vi "AF_Configuration.vi"(1 "ClassRef/ClassPath(If empty Configuration default will be modified)":variant, 5 "Error In":errorcluster) -> (19 "Error Out":errorcluster)   [LabVIEW 2020]
uses:
  LvIcon_class/GDSLvIcon_ColorControl.ctl
  SubVIs/GOOP_WirePattern.ctl
  SubVIs/GOOP_HelpButton.ctl
  SubVIs/GOOP_WireConfigurationType.ctl
  AF_SettingsType.ctl
panel:
  in  "_MessageFolderName":string caption="Virtual message folder name to use"
  in  "_HelpDefaultConfiguration":T1
  in  "_Help":bool
  out "_AFMessageClassItemIconApperance":string caption="Message classes item icon"
  out "_AFWireApperance":string caption="Message class wire Appearance"
  in  "_SetToDefaultForAllClasses":bool caption="Set this to default\nfor all future classes"
  in  "_Cancel":bool
  out "_Preview":picture caption="Preview"
  in  "_Icon":u16(ring) caption="Icon" items=["BlueCircle", "BlueFrame", "BlueFull", "BlueMessage", "BrownCircle", "BrownFrame", "BrownFull", "BurgundyCircle", "BurgundyFrame", "BurgundyFull", "CyanCircle", "CyanFrame", "CyanFull", "DarkBlueCircle", "DarkBlueFrame", "DarkBlueFull", "ForestGreenCircle", "ForestGreenFrame", "ForestGreenFull", "GrayCircle", "GrayFrame", "GrayFull", "GreenCircle", "GreenFrame", "GreenFull", "LightGreenCircle", "LightGreenFrame", "LightGreenFull", "LightRedCircle", "LightRedFrame", "LightRedFull", "PinkCircle", "PinkFrame", "PinkFull", "PurpleCircle", "PurpleFrame", "PurpleFull", "RedCircle", "RedFrame", "RedFull", "YellowCircle", "YellowFrame", "YellowFull"]
  in  "_TunnelsAndTerminalsColors":T2 caption="Tunnels and terminals colors"
  in  "_CenterColor2":T2 caption="Pattern Colors"
  in  "_CenterColor1":T2 caption="Pattern Colors"
  in  "_CenterPattern":T3 caption="Center pattern"
  in  "_EdgeColor":T2 caption="Edge color"
  in  "_CenterThickness":T4(ring) caption="Center thickness"
  in  "_EdgeThickness":T5(ring) caption="Edge thickness"
  out "_AF Message Wire preview":picture caption="Message wire preview"
  in  "_Done":bool
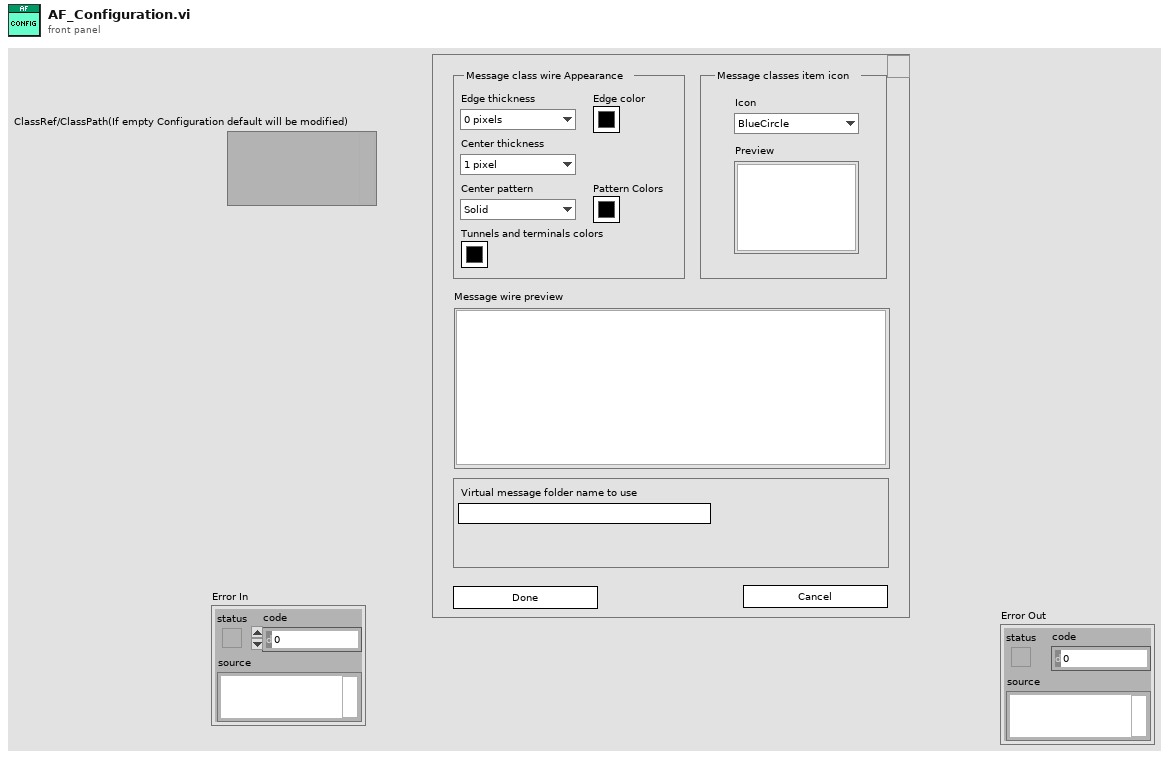
[diagram p1: front panel]
types:
  T1 = typedef "GOOP_HelpButton.ctl" = bool
  T2 = typedef "GDSLvIcon_ColorControl.ctl" = cluster{"Decal":bool, "Color":u32}
  T3 = typedef "GOOP_WirePattern.ctl" = enum16{"Solid", "Large dash", "Small dash"}
  T4 = enum16{"1 pixel", "2 pixels", "3 pixels", "4 pixels", "5 pixels"}
  T5 = enum16{"0 pixels", "1 pixel", "2 pixels", "3 pixels"}
  T6 = cluster{"FirstTime":bool, "ClassRef":refnum<vi>, "ClassRefCreated":bool}
  T7 = typedef "GOOP_WireConfigurationType.ctl" = cluster{"Edge thickness":i32, "Edge color":u32, "Center thickness":i32, "Center pattern":T3, "CenterColor1":u32, "CenterColor2":u32, "Tunnels and terminals colors":u32}
  T8 = typedef "AF_SettingsType.ctl" = cluster{"MessageFolderName":string}
  T9 = cluster{"Foreground Color":u32, "Background Color":u32, "Fill Pattern":cluster{"Row 0":u8, "Row 1":u8, "Row 2":u8, "Row 3":u8, "Row 4":u8, "Row 5":u8, "Row 6":u8, "Row 7":u8}, "Width":i16, "Mode":enum16{"Copy", "Or", "Exclusive Or", "Bit Clear", "Not Copy", "Not Or", "Nor Exclusive Or", "Not Bit Clear"}, "Style":enum32{"Solid", "Dash", "Dot", "Dash Dot", "Dash Dot Dot"}, "Fill Rule":enum32{"Even Odd", "Winding"}, "End Caps":enum32{"Default", "Flat"}}[]
  T10 = typedef "imagedata.ctl" = cluster{"image type":i32, "image depth":i32, "image":u8[], "mask":u8[], "colors":u32[], "Rectangle":cluster{"left":i16, "top":i16, "right":i16, "bottom":i16}}
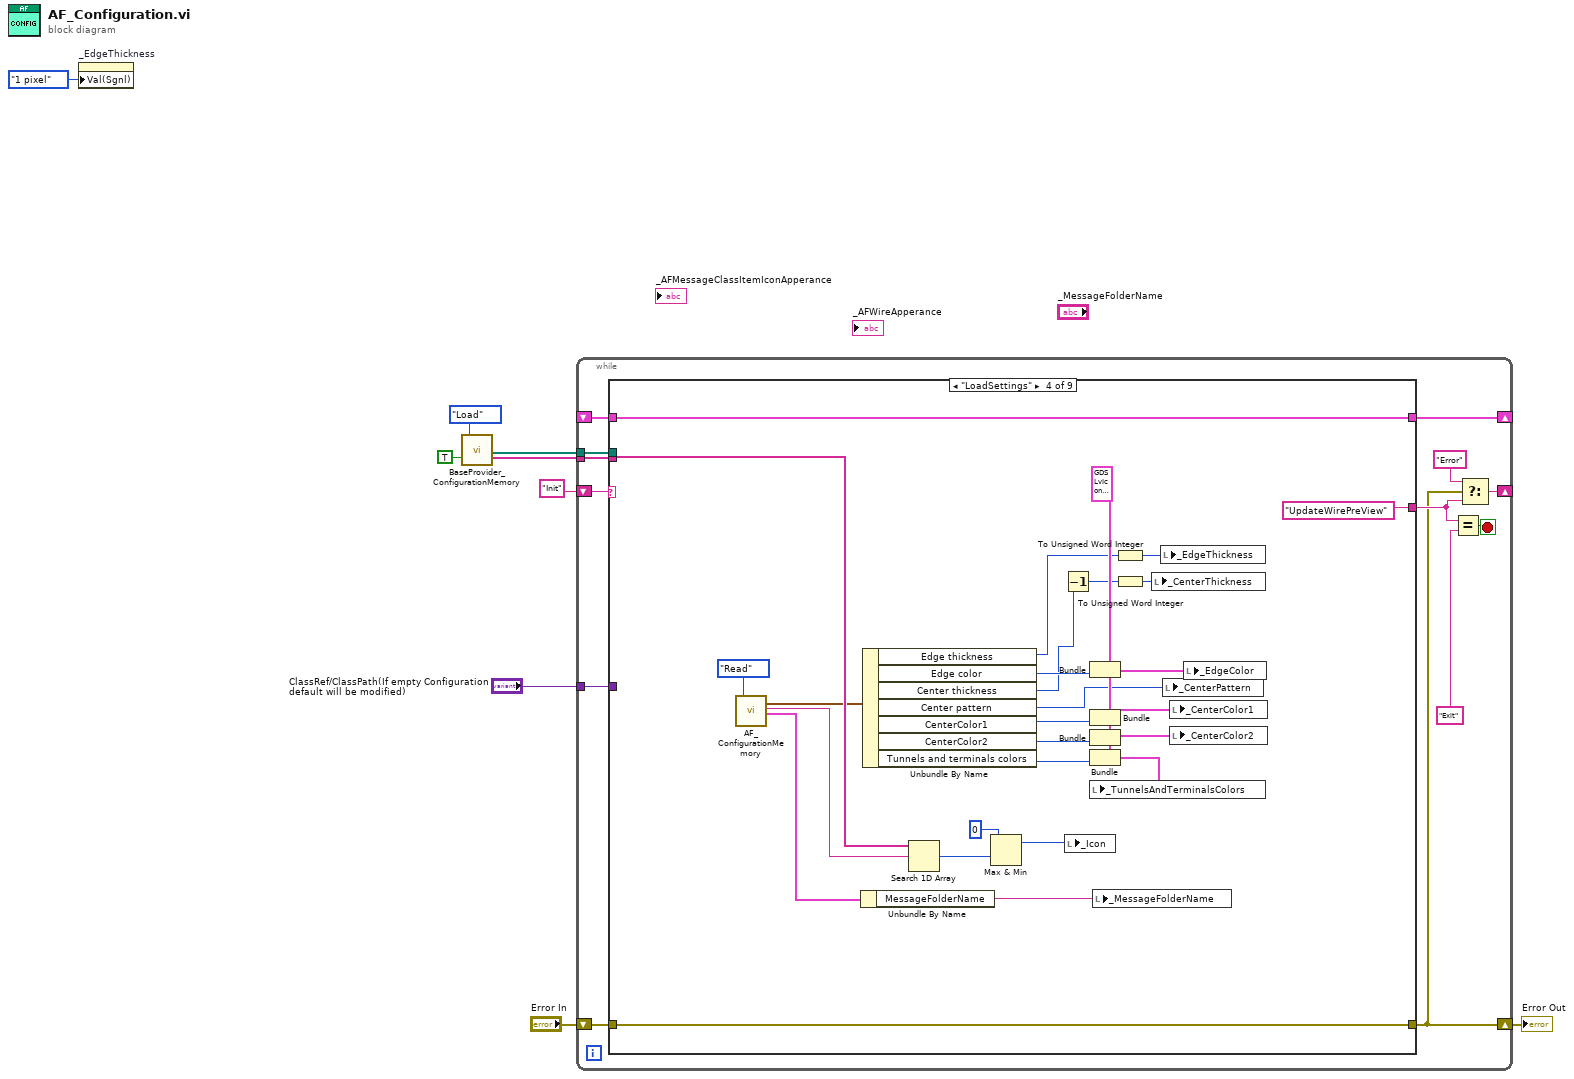
[diagram p0: block diagram]
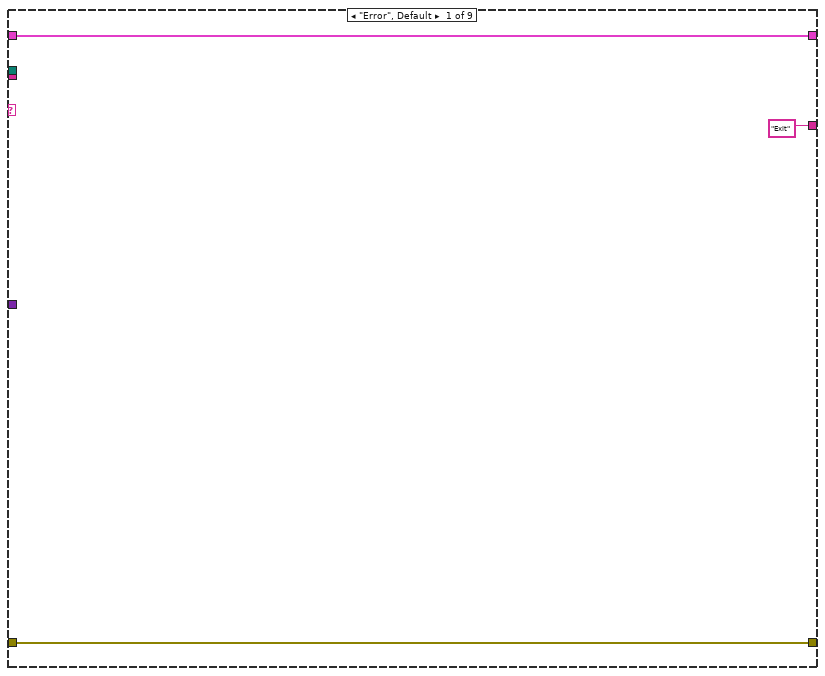
[diagram p2: hidden frame]
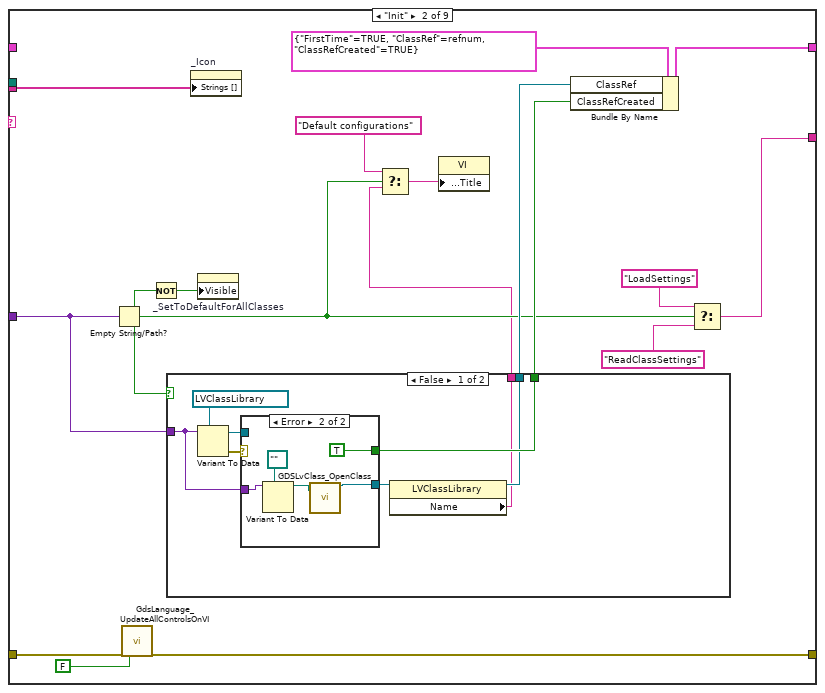
[diagram p3: hidden frame]
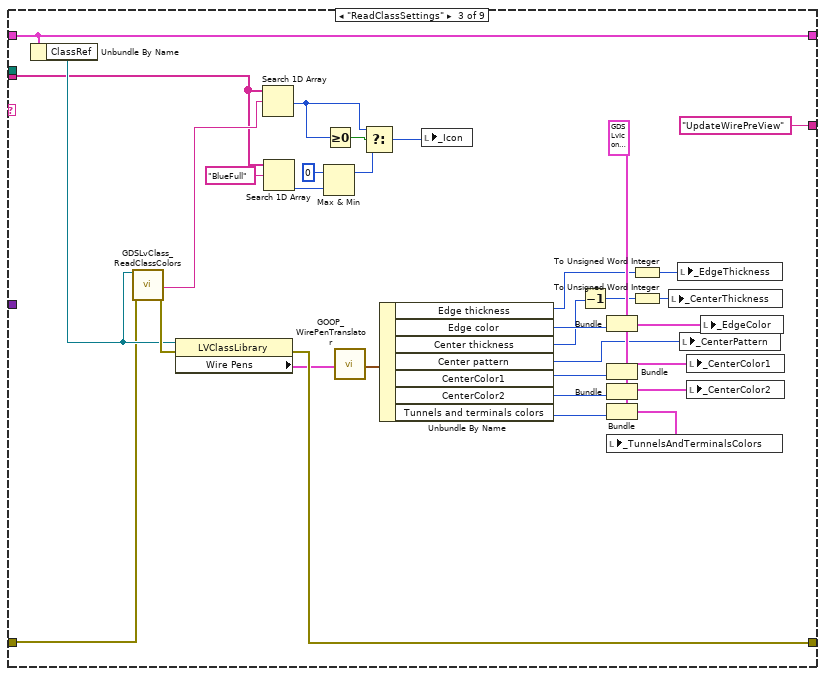
[diagram p6: hidden frame]
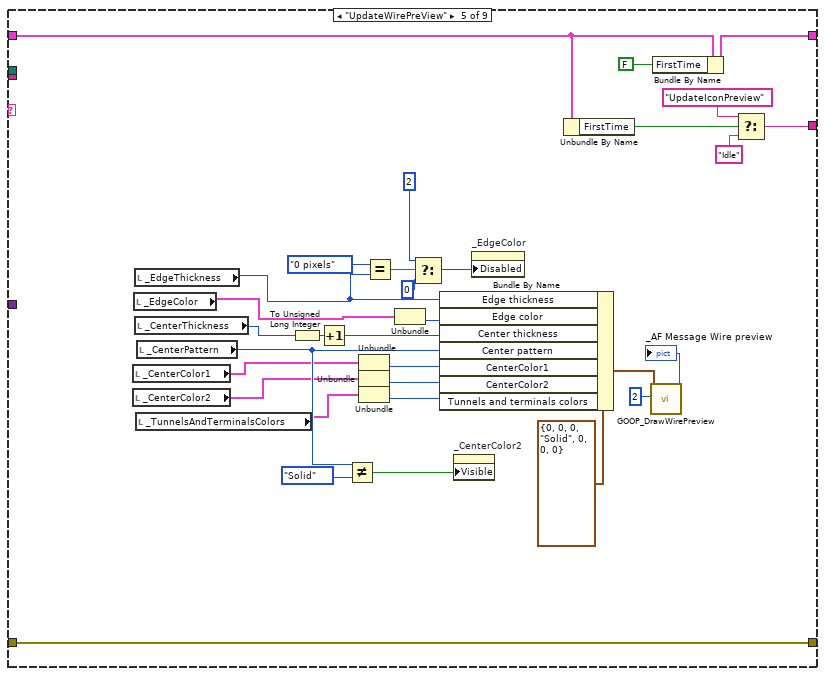
[diagram p7: hidden frame]
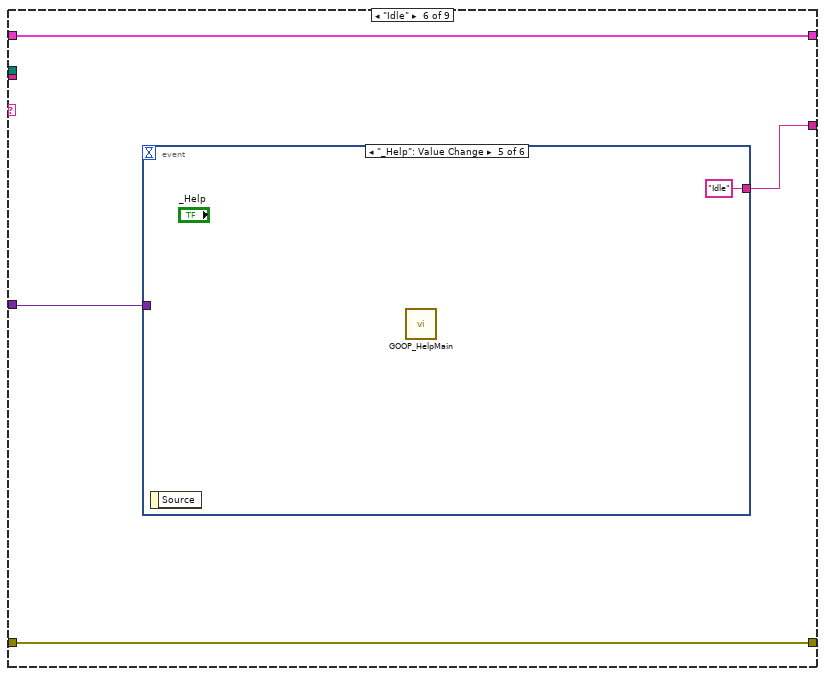
[diagram p8: hidden frame]
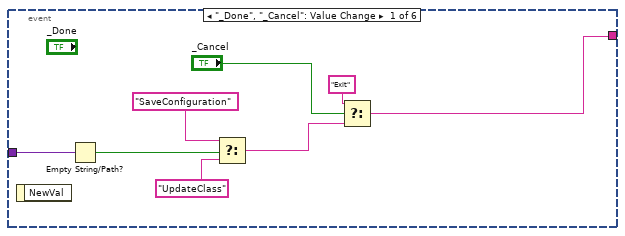
[diagram p9: hidden frame]
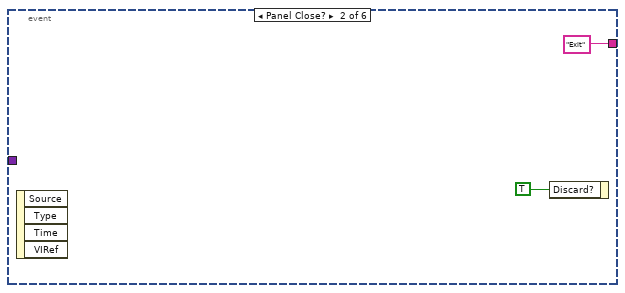
[diagram p10: hidden frame]
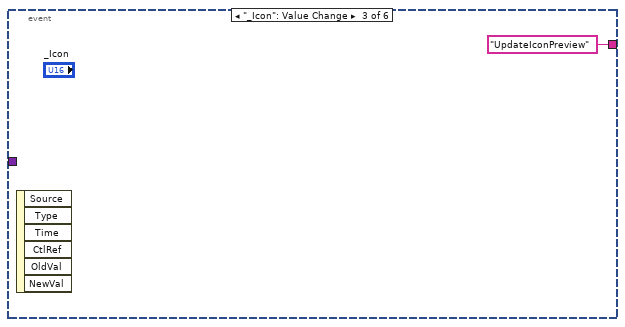
[diagram p11: hidden frame]
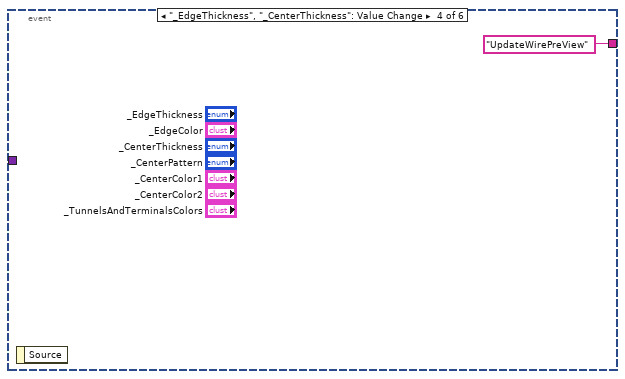
[diagram p12: hidden frame]
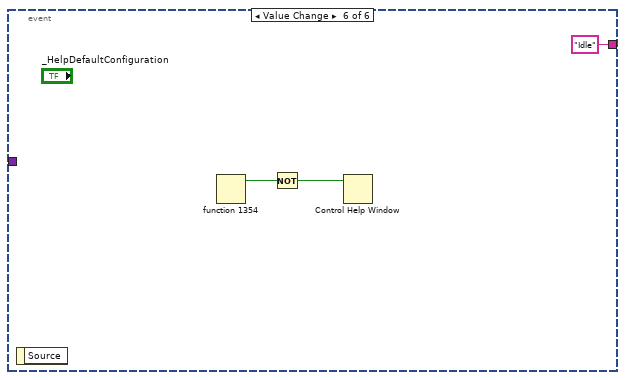
[diagram p13: hidden frame]
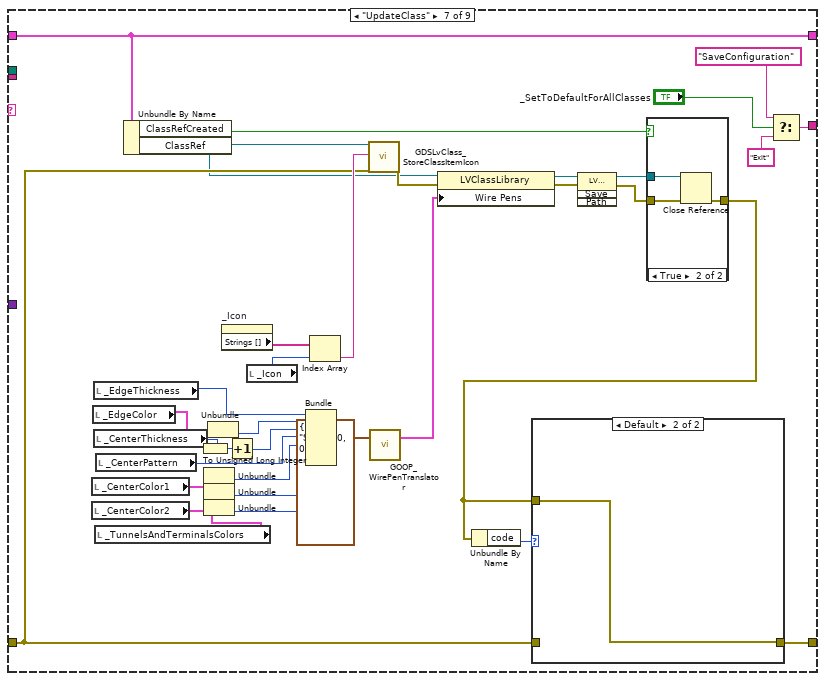
[diagram p14: hidden frame]
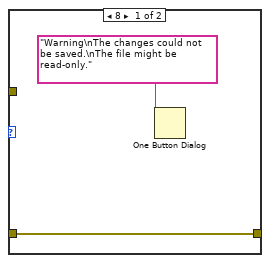
[diagram p15: hidden frame]
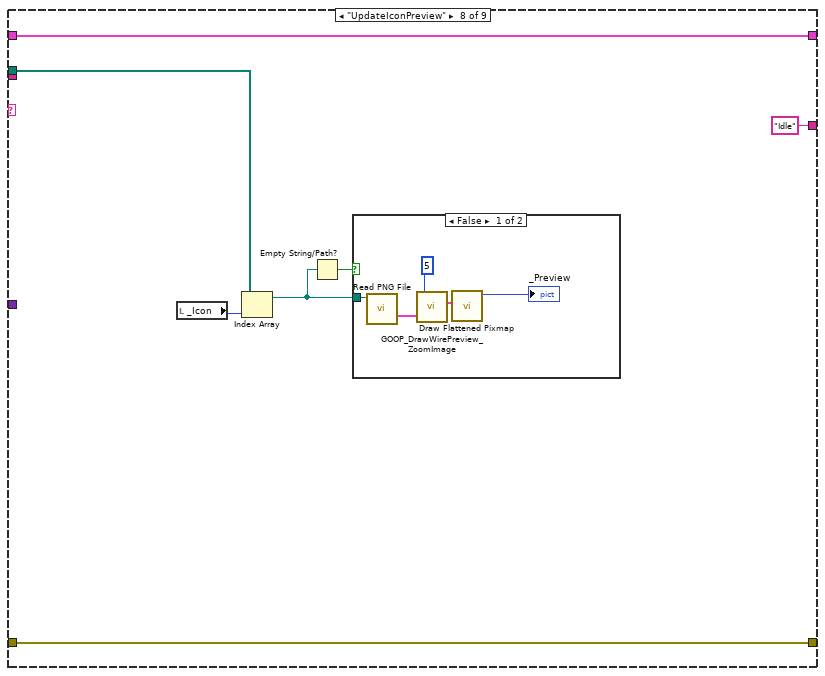
[diagram p17: hidden frame]
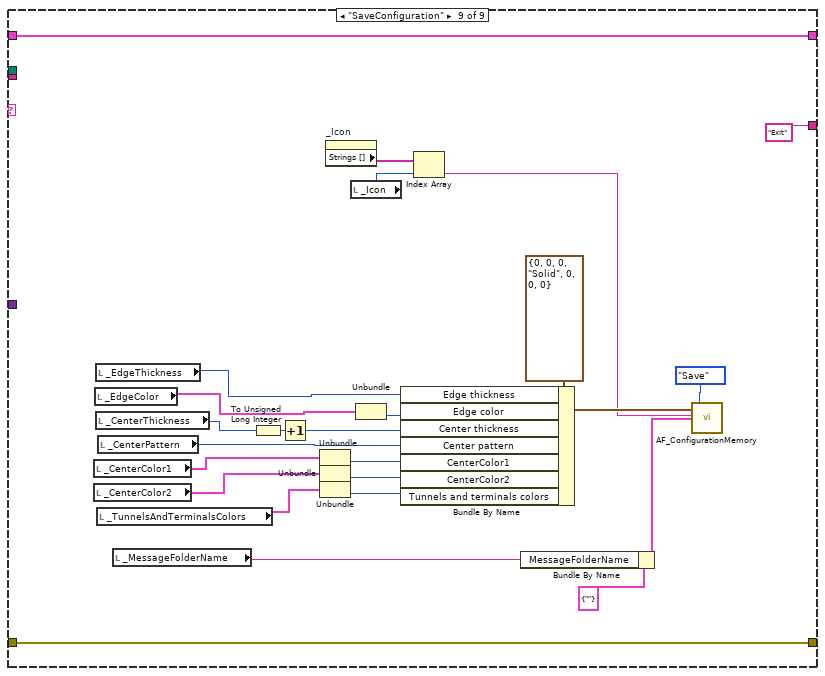
[diagram p19: hidden frame]
diagram:
  n1 = property on="_EdgeThickness" class="Enum (strict)"("Val(Sgnl)"=T5."1 pixel" ("Value (Signaling)")) -> ()  [unwired: 2 in, 2 out]
  n2 = call "BaseProvider_ConfigurationMemory.vi"("Filter_Icons"=TRUE, "Action"=enum16{"Read", "Load", "Save"}."Load") -> ("ClassItemIconPaths"=w1:path[], "ClassItemIconNames"=w2:string[])  [unwired: 11 in, 5 out]
  n3 = while {
    shift-right: [w15] -> w6
    shift-left: "Error In" -> [w22]
    shift-right: [w20] -> _
    shift-left: "Init" -> [w21]
    shift-right: [w14] -> _
    shift-left: _ -> [w13]
    tunnel: "ClassRef/ClassPath(If empty Configuration default will be modified)" -> [w12]
    tunnel: w2 -> [w11]
    tunnel: w1 -> [w10]
    stop <- w19 stop-if-true
    n4 = case shown="\"LoadSettings\"" w21 {
      tunnel: w22 -> [w25 w29 w58 w98 w125 w149 w170 w213 w232]
      tunnel: [w25 w28 w85 w98 w125 w149 w173 w213 w232] -> w15
      tunnel: ["Exit" w41 "UpdateWirePreView" "UpdateWirePreView" w119 w151 w202 "Idle" "Exit"] -> w16
      tunnel: [w23 w35 w88 w99 w124 w150 w197 w215 w230] -> w14
      tunnel: w13 -> [w23 _ w88 w99 w122 w150 w197 w215 w230]
      tunnel: w12 -> [_ w37 _ _ _ w148 _ _ _]
      tunnel: w11 -> [_ w26 w57 w94 _ _ _ _ _]
      tunnel: w10 -> [_ _ _ _ _ _ _ w210 _]
      frame "Error", Default {
      }
      frame "Init" {
        n5 = Empty String/Path?(string/path=w37) -> (empty?=w32:bool)
        n6 = call "GdsLanguage_UpdateAllControlsOnVI.vi"("error in (no error)"=w29, "CreateLanguageFile(Use this to create a languageFile)"=FALSE) -> ("error out"=w28:errorcluster)  [unwired: 16 in, 1 out]
        n7 = Not(x=w32) -> (.not. x?=w31:bool)
        n8 = case shown="False" w32 {
          tunnel: w37 -> [w48 _]
          tunnel: [w44 _] -> w34
          tunnel: [w46 _] -> w33
          tunnel: [w43 _] -> w30
          frame False {
            n9 = Variant To Data(type=refnum<vi> refnum ("Class Refnum In"), Variant=w48) -> (data=w47:refnum<vi>, error out=w49:errorcluster)  [unwired: 1 in]
            n10 = case shown="Error" w49 {
              tunnel: w48 -> [_ w56]
              tunnel: [w51 w53] -> w45
              tunnel: w47 -> [w51 _]
              tunnel: [_ TRUE] -> w46
              frame No Error {
              }
              frame Error {
                n11 = Variant To Data(type=path "", Variant=w56) -> (data=w54:path)  [unwired: 1 in, 1 out]
                n12 = call "GDSLvClass_OpenClass.vi"("ClassToOpen"=w54) -> ("LVClass.Open"=w53:refnum<vi>)  [unwired: 17 in, 1 out]
              }
            }
            n13 = property class="LVClassLibrary"(reference=w45) -> (reference out=w44:refnum<vi>, "Name"=w43:string)  [unwired: 1 in, 1 out]
          }
          frame True {
          }
        }
        n14 = property on="_Icon" class="Ring (strict)"("Strings []"=w26) -> ()  [unwired: 2 in, 2 out]
        n15 = property on="_SetToDefaultForAllClasses" class="Bool (strict)"("Visible"=w31) -> ()  [unwired: 2 in, 2 out]
        n16 = Select(t="Default configurations", s=w32, f=w30) -> (s? t:f=w39:string)
        n17 = property class="VI"("Front Panel.Title"=w39) -> ()  [unwired: 2 in, 2 out]
        n18 = Bundle By Name(cluster=T6 {"FirstTime"=TRUE, "ClassRef"=refnum, "ClassRefCreated"=TRUE}, "ClassRef"=w34, "ClassRefCreated"=w33) -> (w35:T6)
        n19 = Select(t="LoadSettings", s=w32, f="ReadClassSettings") -> (s? t:f=w41:string)
      }
      frame "ReadClassSettings" {
        w77 = T2 {"Decal"=FALSE, "Color"=11184810} ("Edge color")
        n20 = Unbundle By Name(w88) -> ("ClassRef"=w59:refnum<vi>)
        n21 = call "GDSLvClass_ReadClassColors.vi"("Library Refnum"=w59, "error in (no error)"=w58) -> ("ClassItemIconName(NoExtension)"=w84:string, "error out"=w86:errorcluster)  [unwired: 12 in, 4 out]
        n22 = property class="LVClassLibrary"(reference=w59, error in=w86) -> (error out=w85:errorcluster, "Wire Pens"=w83:T9)  [unwired: 1 out]
        n23 = Search 1D Array(1D array=w57, element=w84) -> (index of element=w65:i32)  [unwired: 1 in]
        n24 = Search 1D Array(1D array=w57, element="BlueFull") -> (index of element=w62:i32)  [unwired: 1 in]
        n25 = Max & Min(x=0, y=w62) -> (max(x,y)=w60:i32)  [unwired: 1 out]
        n26 = Greater Or Equal To 0?(x=w65) -> (x >= 0?=w66:bool)
        n27 = call "GOOP_WirePenTranslator.vi"("WirePensIn"=w83) -> ("WireConfigurationOut"=w67:T7)  [unwired: 17 in, 1 out]
        n28 = Select(t=w65, s=w66, f=w60) -> (s? t:f=w64:i32)
        n29 = Unbundle By Name(w67) -> ("Edge thickness"=w69:i32, "Edge color"=w82:u32, "Center thickness"=w72:i32, "Center pattern"=w73:T3, "CenterColor1"=w81:u32, "CenterColor2"=w80:u32, "Tunnels and terminals colors"=w79:u32)
        n30 = local write "_Icon"(w64) -> ()
        n31 = Decrement(x=w72) -> (x-1=w71:i32)
        n32 = Bundle(cluster=w77, "Color"=w82) -> (w74:T2)  [unwired: 1 in]
        n33 = Bundle(cluster=w77, "Color"=w81) -> (w75:T2)  [unwired: 1 in]
        n34 = Bundle(cluster=w77, "Color"=w80) -> (w76:T2)  [unwired: 1 in]
        n35 = Bundle(cluster=w77, "Color"=w79) -> (w78:T2)  [unwired: 1 in]
        n36 = local write "_TunnelsAndTerminalsColors"(w78) -> ()
        n37 = To Unsigned Word Integer(number=w69) -> (unsigned 16bit integer=w68:u16)
        n38 = To Unsigned Word Integer(number=w71) -> (unsigned 16bit integer=w70:u16)
        n39 = local write "_CenterThickness"(w70) -> ()
        n40 = local write "_EdgeThickness"(w68) -> ()
        n41 = local write "_CenterPattern"(w73) -> ()
        n42 = local write "_CenterColor1"(w75) -> ()
        n43 = local write "_CenterColor2"(w76) -> ()
        n44 = local write "_EdgeColor"(w74) -> ()
      }
      frame "LoadSettings" {
        w110 = T2 {"Decal"=FALSE, "Color"=11184810} ("Edge color")
        n45 = call "AF_ConfigurationMemory.vi"("Action"=enum16{"Read", "Load", "Save", "Set"}."Read") -> ("AF_MessaageWireConfigurationOut"=w92:T7, "IconOut"=w91:string, "AF_SettingsOut"=w90:T8)  [unwired: 15 in, 1 out]
        n46 = Unbundle By Name(w90) -> ("MessageFolderName"=w89:string)
        n47 = Unbundle By Name(w92) -> ("Edge thickness"=w102:i32, "Edge color"=w115:u32, "Center thickness"=w105:i32, "Center pattern"=w106:T3, "CenterColor1"=w114:u32, "CenterColor2"=w113:u32, "Tunnels and terminals colors"=w112:u32)
        n48 = Search 1D Array(1D array=w94, element=w91) -> (index of element=w96:i32)  [unwired: 1 in]
        n49 = Max & Min(x=0, y=w96) -> (max(x,y)=w95:i32)  [unwired: 1 out]
        n50 = Decrement(x=w105) -> (x-1=w104:i32)
        n51 = local write "_Icon"(w95) -> ()
        n52 = Bundle(cluster=w110, "Color"=w115) -> (w107:T2)  [unwired: 1 in]
        n53 = Bundle(cluster=w110, "Color"=w114) -> (w108:T2)  [unwired: 1 in]
        n54 = Bundle(cluster=w110, "Color"=w113) -> (w109:T2)  [unwired: 1 in]
        n55 = Bundle(cluster=w110, "Color"=w112) -> (w111:T2)  [unwired: 1 in]
        n56 = local write "_TunnelsAndTerminalsColors"(w111) -> ()
        n57 = local write "_MessageFolderName"(w89) -> ()
        n58 = To Unsigned Word Integer(number=w102) -> (unsigned 16bit integer=w101:u16)
        n59 = To Unsigned Word Integer(number=w104) -> (unsigned 16bit integer=w103:u16)
        n60 = local write "_CenterThickness"(w103) -> ()
        n61 = local write "_EdgeThickness"(w101) -> ()
        n62 = local write "_CenterPattern"(w106) -> ()
        n63 = local write "_CenterColor1"(w108) -> ()
        n64 = local write "_CenterColor2"(w109) -> ()
        n65 = local write "_EdgeColor"(w107) -> ()
      }
      frame "UpdateWirePreView" {
        n66 = local read "_CenterColor1"() -> (w128:T2)
        n67 = local read "_CenterColor2"() -> (w127:T2)
        n68 = local read "_EdgeColor"() -> (w131:T2)
        n69 = local read "_EdgeThickness"() -> (w132:T5)
        n70 = local read "_CenterThickness"() -> (w130:T4)
        n71 = local read "_TunnelsAndTerminalsColors"() -> (w126:T2)
        n72 = local read "_CenterPattern"() -> (w129:T3)
        n73 = To Unsigned Long Integer(number=w130) -> (unsigned 32bit integer=w147:u32)
        n74 = Increment(x=w147) -> (x+1=w140:u32)
        n75 = Not Equal?(x=w129, y=GOOP_WirePattern."Solid") -> (x != y?=w117:bool)
        n76 = Unbundle(w128) -> ("Color"=w138:u32)  [unwired: 1 out]
        n77 = Unbundle(w127) -> ("Color"=w139:u32)  [unwired: 1 out]
        n78 = Unbundle(w126) -> ("Color"=w136:u32)  [unwired: 1 out]
        n79 = Equal?(x=T5."0 pixels", y=w132) -> (x = y?=w142:bool)
        n80 = Unbundle(w131) -> ("Color"=w137:u32)  [unwired: 1 out]
        n81 = Select(t=u8 2 ("Disabled"), s=w142, f=u8 0) -> (s? t:f=w144:u8)
        n82 = Bundle By Name(cluster=T7 {"Edge thickness"=0, "Edge color"=0, "Center thickness"=0, "Center pattern"=enum."Solid", "CenterColor1"=0, "CenterColor2"=0, "Tunnels and terminals colors"=0} ("WireConfiguration"), "Edge thickness"=w132, "Edge color"=w137, "Center thickness"=w140, "Center pattern"=w129, "CenterColor1"=w138, "CenterColor2"=w139, "Tunnels and terminals colors"=w136) -> (w116:T7)
        n83 = property on="_CenterColor2" class="Clust (strict)"("Visible"=w117) -> ()  [unwired: 2 in, 2 out]
        n84 = property on="_EdgeColor" class="Clust (strict)"("Disabled"=w144) -> ()  [unwired: 2 in, 2 out]
        n85 = Unbundle By Name(w122) -> ("FirstTime"=w121:bool)
        n86 = call "GOOP_DrawWirePreview.vi"("WireConfiguration"=w116, "Zoom"=2) -> ("Picture"=→"_AF Message Wire preview":picture)  [unwired: 16 in, 1 out]
        n87 = Bundle By Name(cluster=w122, "FirstTime"=FALSE) -> (w124:T6)
        n88 = Select(t="UpdateIconPreview", s=w121, f="Idle") -> (s? t:f=w119:string)
      }
      frame "Idle" {
        n89 = event shown="[4] \"_Help\": Value Change" {
          selector: _ -> [_ _ _ _ _ _]
          dyn-events: _ -> [_ _ _ _ _ _]
          timeout: _ -> [_ _ _ _ _ _]
          tunnel: [w153 "Exit" "UpdateIconPreview" "UpdateWirePreView" "Idle" "Idle"] -> w151
          tunnel: w148 -> [w159 _ _ _ _ _]
          event "_Done", "_Cancel": Value Change {
            n90 = event-data() -> ()  [unwired: 1 in, 1 out]
            n91 = Empty String/Path?(string/path=w159) -> (empty?=w158:bool)
            n92 = Select(t="SaveConfiguration", s=w158, f="UpdateClass") -> (s? t:f=w154:string)
            n93 = Select(t="Exit", s="_Cancel", f=w154) -> (s? t:f=w153:string)
          }
          event Panel Close? {
            n94 = event-data() -> ()  [unwired: 1 in, 4 out]
            n95 = event-data("Discard?"=TRUE) -> ()  [unwired: 1 in, 1 out]
          }
          event "_Icon": Value Change {
            n96 = event-data() -> ()  [unwired: 1 in, 6 out]
          }
          event "_EdgeThickness", "_CenterThickness": Value Change {
            n97 = event-data() -> ()  [unwired: 1 in, 1 out]
          }
          event "_Help": Value Change {
            n98 = event-data() -> ()  [unwired: 1 in, 1 out]
            n99 = call "GOOP_HelpMain.vi"() -> ()  [unwired: 12 in]
          }
          event Value Change {
            n100 = event-data() -> ()  [unwired: 1 in, 1 out]
            n101 = fn#1354() -> (1:w166:bool)  [unwired: 1 out]
            n102 = Not(x=w166) -> (.not. x?=w165:bool)
            n103 = Control Help Window(1:w165) -> ()  [unwired: 1 in]
          }
        }
      }
      frame "UpdateClass" {
        n104 = local read "_CenterColor1"() -> (w183:T2)
        n105 = local read "_CenterColor2"() -> (w187:T2)
        n106 = local read "_EdgeColor"() -> (w185:T2)
        n107 = local read "_EdgeThickness"() -> (w189:T5)
        n108 = local read "_CenterThickness"() -> (w184:T4)
        n109 = local read "_TunnelsAndTerminalsColors"() -> (w182:T2)
        n110 = local read "_CenterPattern"() -> (w192:T3)
        n111 = Unbundle By Name(w197) -> ("ClassRefCreated"=w199:bool, "ClassRef"=w169:refnum<vi>)
        n112 = To Unsigned Long Integer(number=w184) -> (unsigned 32bit integer=w186:u32)
        n113 = Unbundle(w183) -> ("Color"=w193:u32)  [unwired: 1 out]
        n114 = Unbundle(w187) -> ("Color"=w194:u32)  [unwired: 1 out]
        n115 = Unbundle(w182) -> ("Color"=w195:u32)  [unwired: 1 out]
        n116 = Unbundle(w185) -> ("Color"=w190:u32)  [unwired: 1 out]
        n117 = property on="_Icon" class="Ring (strict)"() -> ("Strings []"=w180:string[])  [unwired: 2 in, 2 out]
        n118 = Increment(x=w186) -> (x+1=w191:u32)
        n119 = local read "_Icon"() -> (w179:u16)
        n120 = Bundle(cluster=T7 {"Edge thickness"=0, "Edge color"=0, "Center thickness"=0, "Center pattern"=enum."Solid", "CenterColor1"=0, "CenterColor2"=0, "Tunnels and terminals colors"=0} ("WireConfiguration"), "Edge thickness"=w189, "Edge color"=w190, "Center thickness"=w191, "Center pattern"=w192, "CenterColor1"=w193, "CenterColor2"=w194, "Tunnels and terminals colors"=w195) -> (w181:T7)
        n121 = Index Array(array=w180, index=w179) -> (element=w175:string)
        n122 = call "GDSLvClass_StoreClassItemIcon.vi"("Library Refnum"=w169, "ClassItemIconName"=w175, "error in (no error)"=w170) -> ("error out"=w171:errorcluster)  [unwired: 15 in, 1 out]
        n123 = call "GOOP_WirePenTranslator.vi"("WireConfigurationIn"=w181) -> ("WirePensOut"=w196:T9)  [unwired: 17 in, 1 out]
        n124 = property class="LVClassLibrary"(reference=w169, error in=w171, "Wire Pens"=w196) -> (reference out=w178:refnum<vi>, error out=w177:errorcluster)
        n125 = invoke class="LVClassLibrary" method="Save"(reference=w178, error in=w177) -> (reference out=w176:refnum<vi>, error out=w168:errorcluster)  [unwired: 2 in, 2 out]
        n126 = case shown="True" w199 {
          tunnel: w168 -> [w206 w209]
          tunnel: w176 -> [_ w208]
          tunnel: [w206 w207] -> w172
          frame False {
          }
          frame True {
            n127 = Close Reference(reference=w208, error in (no error)=w209) -> (error out=w207:errorcluster)
          }
        }
        n128 = Unbundle By Name(w172) -> ("code"=w174:i32)
        n129 = case shown="Default" w174 {
          tunnel: w170 -> [w203 _]
          tunnel: [w203 w205] -> w173
          tunnel: w172 -> [_ w205]
          frame 8 {
            n130 = One Button Dialog(message="Warning\nThe changes could not be saved.\nThe file might be read-only.") -> ()  [unwired: 1 in, 1 out]
          }
          frame Default {
          }
        }
        n131 = Select(t="SaveConfiguration", s="_SetToDefaultForAllClasses", f="Exit") -> (s? t:f=w202:string)
      }
      frame "UpdateIconPreview" {
        n132 = local read "_Icon"() -> (w214:u16)
        n133 = Index Array(array=w210, index=w214) -> (element=w212:path)
        n134 = Empty String/Path?(string/path=w212) -> (empty?=w211:bool)
        n135 = case shown="False" w211 {
          tunnel: w212 -> [w217 _]
          frame False {
            n136 = call <vilib>:"Read PNG File.vi"("path to PNG file"=w217) -> ("image data"=w220:T10)  [unwired: 8 in, 2 out]
            n137 = call "GOOP_DrawWirePreview_ZoomImage.vi"("image data 2"=w220, "Zoom"=5) -> ("image data"=w221:T10)
            n138 = call <vilib>:"Draw Flattened Pixmap.vi"("image data"=w221) -> ("new picture"=→"_Preview":picture)  [unwired: 8 in]
          }
          frame True {
          }
        }
      }
      frame "SaveConfiguration" {
        n139 = local read "_CenterColor1"() -> (w235:T2)
        n140 = local read "_CenterColor2"() -> (w234:T2)
        n141 = local read "_EdgeColor"() -> (w238:T2)
        n142 = local read "_EdgeThickness"() -> (w239:T5)
        n143 = local read "_CenterThickness"() -> (w237:T4)
        n144 = local read "_TunnelsAndTerminalsColors"() -> (w233:T2)
        n145 = local read "_CenterPattern"() -> (w236:T3)
        n146 = local read "_MessageFolderName"() -> (w223:string)
        n147 = To Unsigned Long Integer(number=w237) -> (unsigned 32bit integer=w246:u32)
        n148 = Increment(x=w246) -> (x+1=w245:u32)
        n149 = Unbundle(w235) -> ("Color"=w243:u32)  [unwired: 1 out]
        n150 = Unbundle(w234) -> ("Color"=w244:u32)  [unwired: 1 out]
        n151 = Unbundle(w233) -> ("Color"=w241:u32)  [unwired: 1 out]
        n152 = property on="_Icon" class="Ring (strict)"() -> ("Strings []"=w229:string[])  [unwired: 2 in, 2 out]
        n153 = local read "_Icon"() -> (w228:u16)
        n154 = Unbundle(w238) -> ("Color"=w242:u32)  [unwired: 1 out]
        n155 = Bundle By Name(cluster=T7 {"Edge thickness"=0, "Edge color"=0, "Center thickness"=0, "Center pattern"=enum."Solid", "CenterColor1"=0, "CenterColor2"=0, "Tunnels and terminals colors"=0} ("WireConfiguration"), "Edge thickness"=w239, "Edge color"=w242, "Center thickness"=w245, "Center pattern"=w236, "CenterColor1"=w243, "CenterColor2"=w244, "Tunnels and terminals colors"=w241) -> (w226:T7)
        n156 = Index Array(array=w229, index=w228) -> (element=w225:string)
        n157 = Bundle By Name(cluster=T8 {"MessageFolderName"=""} ("AF_Settings"), "MessageFolderName"=w223) -> (w222:T8)
        n158 = call "AF_ConfigurationMemory.vi"("AF_MessaageWireConfiguration"=w226, "Icon"=w225, "AF_Settings"=w222, "Action"=enum16{"Read", "Load", "Save", "Set"}."Save") -> ()  [unwired: 12 in, 4 out]
      }
    }
    n159 = Equal?(x=w16, y="Exit") -> (x = y?=w19:bool)
    n160 = Select(t="Error", s=w15, f=w16) -> (s? t:f=w20:string)
  }
  "Error Out" <- w6
